vi "Open_COM.vi"(0 "USB-87Pn in":refnum<class "USB-87Pn.lvclass">, 1 "port number":u8=1, 5 "baudrate (115200)":u32=115200, 7 "data bit (8)":u8=8, 9 "stop bit (0: 1 stop bit)":u8(ring) items=["1 stop bit", "1.5 stop bit", "2 stop bit"], 11 "error in (no error)":errorcluster, 12 "parity (0: none)":u8(ring) items=["none parity", "odd parity", "even parity"]) -> (4 "USB-87Pn out":refnum<class "USB-87Pn.lvclass">, 15 "error out":errorcluster)   [LabVIEW 2019, in "USB-87Pn.lvlib" / "USB-87Pn.lvclass"]
uses:
  USB-87Pn.lvclass
  USB-87Pn.lvclass/USB-87Pn.ctl
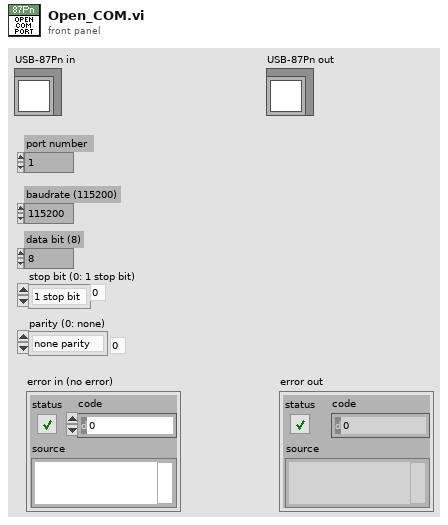
[diagram p1: front panel]
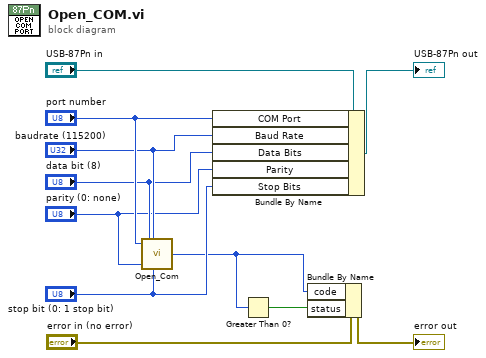
[diagram p0: block diagram]
diagram:
  n1 = call <vilib>:"Open_Com.VI"("port number"="port number", "baudrate (115200)"="baudrate (115200)", "data bit (8)"="data bit (8)", "parity (0: none)"="parity (0: none)", "stop bit (0: 1 stop bit)"="stop bit (0: 1 stop bit)") -> ("return"=w2:u16)
  n2 = Bundle By Name(cluster="USB-87Pn in", "COM Port"="port number", "Baud Rate"="baudrate (115200)", "Data Bits"="data bit (8)", "Parity"="parity (0: none)", "Stop Bits"="stop bit (0: 1 stop bit)") -> (→"USB-87Pn out":refnum<class "USB-87Pn.lvclass">)
  n3 = Greater Than 0?(x=w2) -> (x > 0?=w1:bool)
  n4 = Bundle By Name(cluster="error in (no error)", "code"=w2, "status"=w1) -> (→"error out":errorcluster)
